vi "IDE_msg_Example_new.vi"() -> ()   [LabVIEW 2020]
uses:
  LabVIEWCode/Subs/ColorText/Code.xctl
  LabVIEWCode/Subs/Console XCtrl/Console_Xctrl.xctl
  LabVIEWCode/Subs/Server XCtrl/Server.xctl
panel:
  in  "Clean":bool
  in  "PC Save":bool
  in  "PC path":path=path "/Users/milandahal/Documents/GitHub/Summer2020/MilanTest/request.py"
  in  "Files":bool
  in  "Server":bool
  in  "Help":bool
  in  "Server":path(xcontrol)=path "/Users/milandahal/Documents/GitHub/Summer2020/LabVIEWCode/Servers/Jens.vi"
  out "REPL":string(xcontrol)="\nTraceback (most recent call last):\n  File \"<stdin>\", line 1\nSyntaxError: invalid syntax\n>>> import hub,utime, ujson\n>>> class request:\n...     def __init__(self):\n...         self.ser = hub.USB_VCP()\n...         self.mbegin=b'msg_start\\n'\n...         self.mend=b'\\nmsg_end\\n'\n...         self.rbegin = b'reply_start '\n...         self.rend = b' reply_end'\n...     def comm(self,payload):\n...         s =  b' '\n...         self.ser.write(self.mbegin + payload + self.mend)\n...         utime.sleep(0.01)\n...         while not(rend in s):\n...             try:\n...                 s = s + self.ser.readline()\n...             except:\n...                 utime.sleep(0.1)\n...         start = len(self.rbegin)+s.find(self.rbegin)\n...         end = s.find(self.rend)\n...         reply = s[start:end]\n...         return reply.decode()\n...     def put(self, headers, url, data):\n...         request= {\"method\": \"put\",\"headers\": ujson.dumps(headers) ,\"url\": url,\"data\": ujson.dumps(data) }\n...         reply=comm(ujson.dumps(request))\n...         utime.sleep(01)\n...         return(reply)        \n...     def post(self, headers, url, data):\n...         request= {\"method\": \"post\",\"headers\": ujson.dumps(headers) ,\"url\": url,\"data\": ujson.dumps(data) }\n...         reply=comm(ujson.dumps(request))\n...         utime.sleep(01)\n...         return(reply)  \n...     def get(self, headers , url):\n...         request= {\"method\": \"get\",\"headers\": ujson.dumps(headers) ,\"url\": url}\n...         reply=comm(ujson.dumps(request))\n...         utime.sleep(01)\n...         return(reply)\n... \n>>> test=request()\n>>> SL_Appkey= \"bvd8X9LweQY9o2eP1NYL-p8mLL9wMAk6YYOnYSiIo0\" \n>>> Headers={\"Accept\":\"application/json\",\"x-ni-api-key\": SL_Appkey }\n>>> Url=\"https://api.systemlinkcloud.com/nitag/v2/tags/test1/values/current\"\n>>> Data={\"value\":{\"type\":\"STRING\",\"value\":\"lol\"}}\n>>> print(reply1)\n{\"timestamp\":\"2020-06-05T14:56:55.375191Z\",\"value\":{\"type\":\"STRING\",\"value\":\"lol\"}}\n>>> key = \"b6fb6cd636d2c3f44a1f7949ff4febf7\"\n>>> city_id = \"7872695\" \n>>> baseurl = \"https://api.openweathermap.org/\"\n>>> url = baseurl + \"data/2.5/weather?id=\" + city_id + \"&appid=\" + key\n>>> reply3= test.get(headers={}, url=url)\nmsg_start\n{\"url\": \"https://api.openweathermap.org/data/2.5/weather?id=7872695&appid=b6fb6cd636d2c3f44a1f7949ff4febf7\", \"headers\": \"{}\", \"method\": \"get\"}\nmsg_end\nb' \\n'\nb' \\nreply_start {\"coord\":{\"lon\":16.21,\"lat\":47.19},\"weather\":[{\"id\":804,\"main\":\"Clouds\",\"description\":\"overcast clouds\",\"icon\":\"04d\"}],\"base\":\"stations\",\"main\":{\"temp\":289.53,\"feels_like\":290.97,\"temp_min\":289.26,\"temp_max\":289.82,\"pressure\":1001,\"humidity\":94},\"wind\":{\"speed\":0.46,\"deg\":71},\"clouds\":{\"all\":100},\"dt\":1591370040,\"sys\":{\"type\":3,\"id\":2007196,\"country\":\"AT\",\"sunrise\":1591326068,\"sunset\":1591382795},\"timezone\":7200,\"id\":7872695,\"name\":\"Olbendorf\",\"cod\":200} reply_end'\n>>> reply_start {\"coord\":{\"lon\":16.21,\"lat\":47.19},\"weather\":[{\"id\":804,\"main\":\"Clouds\",\"description\":\"overcast clouds\",\"icon\":\"04d\"}],\"base\":\"stations\",\"main\":{\"temp\":289.53,\"feels_like\":290.97,\"temp_min\":289.26,\"temp_max\":289.82,\"pressure\":1001,\"humidity\":94},\"wind\":{\"speed\":0.46,\"deg\":71},\"clouds\":{\"all\":100},\"dt\":1591370040,\"sys\":{\"type\":3,\"id\":2007196,\"country\":\"AT\",\"sunrise\":1591326068,\"sunset\":1591382795},\"timezone\":7200,\"id\":7872695,\"name\":\"Olbendorf\",\"cod\":200} reply_end\nTraceback (most recent call last):\n  File \"<stdin>\", line 1\nSyntaxError: invalid syntax\n>>> \n>>> print(reply3)\n{\"coord\":{\"lon\":16.21,\"lat\":47.19},\"weather\":[{\"id\":804,\"main\":\"Clouds\",\"description\":\"overcast clouds\",\"icon\":\"04d\"}],\"base\":\"stations\",\"main\":{\"temp\":289.53,\"feels_like\":290.97,\"temp_min\":289.26,\"temp_max\":289.82,\"pressure\":1001,\"humidity\":94},\"wind\":{\"speed\":0.46,\"deg\":71},\"clouds\":{\"all\":100},\"dt\":1591370040,\"sys\":{\"type\":3,\"id\":2007196,\"country\":\"AT\",\"sunrise\":1591326068,\"sunset\":1591382795},\"timezone\":7200,\"id\":7872695,\"name\":\"Olbendorf\",\"cod\":200}\n>>> import hub,utime, ujson\n>>> class request:\n...     def __init__(self):\n...         self.ser = hub.USB_VCP()\n...         self.mbegin=b'msg_start\\n'\n...         self.mend=b'\\nmsg_end\\n'\n...         self.rbegin = b'reply_start '\n...         self.rend = b' reply_end'\n...     def comm(self,payload):\n...         s =  b' '\n...         self.ser.write(self.mbegin + payload + self.mend)\n...         utime.sleep(0.01)\n...         while not(rend in s):\n...             try:\n...                 s = s + self.ser.readline()\n...             except:\n...                 utime.sleep(0.1)\n...         start = len(self.rbegin)+s.find(self.rbegin)\n...         end = s.find(self.rend)\n...         reply = s[start:end]\n...         return reply.decode()\n...     def put(self, headers, url, data):\n...         request= {\"method\": \"put\",\"headers\": ujson.dumps(headers) ,\"url\": url,\"data\": ujson.dumps(data) }\n...         reply=comm(ujson.dumps(request))\n...         utime.sleep(01)\n...         return(reply)        \n...     def post(self, headers, url, data):\n...         request= {\"method\": \"post\",\"headers\": ujson.dumps(headers) ,\"url\": url,\"data\": ujson.dumps(data) }\n...         reply=comm(ujson.dumps(request))\n...         utime.sleep(01)\n...         return(reply)  \n...     def get(self, headers , url):\n...         request= {\"method\": \"get\",\"headers\": ujson.dumps(headers) ,\"url\": url}\n...         reply=comm(ujson.dumps(request))\n...         utime.sleep(01)\n...         return(reply)\n... \n>>> test=request()\n>>> SL_Appkey= \"bvd8X9LweQY9o2eP1NYL-p8mLL9wMAk6YYOnYSiIo0\" \n>>> Headers={\"Accept\":\"application/json\",\"x-ni-api-key\": SL_Appkey }\n>>> Url=\"https://api.systemlinkcloud.com/nitag/v2/tags/test1/values/current\"\n>>> Data={\"value\":{\"type\":\"STRING\",\"value\":\"lol\"}}\n>>> print(reply1)\n{\"timestamp\":\"2020-06-05T14:56:55.375191Z\",\"value\":{\"type\":\"STRING\",\"value\":\"lol\"}}\n>>> key = \"b6fb6cd636d2c3f44a1f7949ff4febf7\"\n>>> city_id = \"7872695\" \n>>> baseurl = \"https://api.openweathermap.org/\"\n>>> url = baseurl + \"data/2.5/weather?id=\" + city_id + \"&appid=\" + key\n>>> reply3= test.get(headers={}, url=url)\nmsg_start\n{\"url\": \"https://api.openweathermap.org/data/2.5/weather?id=7872695&appid=b6fb6cd636d2c3f44a1f7949ff4febf7\", \"headers\": \"{}\", \"method\": \"get\"}\nmsg_end\nb' \\n'\nb' \\nreply_start {\"coord\":{\"lon\":16.21,\"lat\":47.19},\"weather\":[{\"id\":804,\"main\":\"Clouds\",\"description\":\"overcast clouds\",\"icon\":\"04d\"}],\"base\":\"stations\",\"main\":{\"temp\":289.53,\"feels_like\":290.97,\"temp_min\":289.26,\"temp_max\":289.82,\"pressure\":1001,\"humidity\":94},\"wind\":{\"speed\":0.46,\"deg\":71},\"clouds\":{\"all\":100},\"dt\":1591370040,\"sys\":{\"type\":3,\"id\":2007196,\"country\":\"AT\",\"sunrise\":1591326068,\"sunset\":1591382795},\"timezone\":7200,\"id\":7872695,\"name\":\"Olbendorf\",\"cod\":200} reply_end'\n>>> reply_start {\"coord\":{\"lon\":16.21,\"lat\":47.19},\"weather\":[{\"id\":804,\"main\":\"Clouds\",\"description\":\"overcast clouds\",\"icon\":\"04d\"}],\"base\":\"stations\",\"main\":{\"temp\":289.53,\"feels_like\":290.97,\"temp_min\":289.26,\"temp_max\":289.82,\"pressure\":1001,\"humidity\":94},\"wind\":{\"speed\":0.46,\"deg\":71},\"clouds\":{\"all\":100},\"dt\":1591370040,\"sys\":{\"type\":3,\"id\":2007196,\"country\":\"AT\",\"sunrise\":1591326068,\"sunset\":1591382795},\"timezone\":7200,\"id\":7872695,\"name\":\"Olbendorf\",\"cod\":200} reply_end\nTraceback (most recent call last):\n  File \"<stdin>\", line 1\nSyntaxError: invalid syntax\n>>> print(reply3)\n{\"coord\":{\"lon\":16.21,\"lat\":47.19},\"weather\":[{\"id\":804,\"main\":\"Clouds\",\"description\":\"overcast clouds\",\"icon\":\"04d\"}],\"base\":\"stations\",\"main\":{\"temp\":289.53,\"feels_like\":290.97,\"temp_min\":289.26,\"temp_max\":289.82,\"pressure\":1001,\"humidity\":94},\"wind\":{\"speed\":0.46,\"deg\":71},\"clouds\":{\"all\":100},\"dt\":1591370040,\"sys\":{\"type\":3,\"id\":2007196,\"country\":\"AT\",\"sunrise\":1591326068,\"sunset\":1591382795},\"timezone\":7200,\"id\":7872695,\"name\":\"Olbendorf\",\"cod\":200}\n>>> print(\"something\") \nsomething\n>>> "
  in  "Clear":bool
  in  "Save":bool
  in  "Stop":bool
  in  "Run":bool
  in  "Name":string="code.py"
  in  "Code":string(xcontrol)="import hub,utime, ujson\n\n\n\nclass request:\n    def __init__(self):\n        self.ser = hub.USB_VCP()\n        self.mbegin=b'msg_start\\n'\n        self.mend=b'\\nmsg_end\\n'\n        self.rbegin = b'reply_start '\n        self.rend = b' reply_end'\n    \n    def comm(self,payload):\n        s =  b' '\n        self.ser.write(self.mbegin + payload + self.mend)\n        utime.sleep(0.01)\n        while not(rend in s):\n            try:\n                s = s + self.ser.readline()\n                # print(s)   \n            except:\n                utime.sleep(0.1)\n        start = len(self.rbegin)+s.find(self.rbegin)\n        end = s.find(self.rend)\n        reply = s[start:end]\n        \n        return reply.decode()\n    def put(self, headers, url, data):\n        request= {\"method\": \"put\",\"headers\": ujson.dumps(headers) ,\"url\": url,\"data\": ujson.dumps(data) }\n        reply=comm(ujson.dumps(request))\n        utime.sleep(01)\n        return(reply)        \n    def post(self, headers, url, data):\n        request= {\"method\": \"post\",\"headers\": ujson.dumps(headers) ,\"url\": url,\"data\": ujson.dumps(data) }\n        reply=comm(ujson.dumps(request))\n        utime.sleep(01)\n        return(reply)  \n        \n    def get(self, headers , url):\n        request= {\"method\": \"get\",\"headers\": ujson.dumps(headers) ,\"url\": url}\n        reply=comm(ujson.dumps(request))\n        utime.sleep(01)\n        return(reply)\n        \n\ntest=request()\nSL_Appkey= \"bvd8X9LweQY9o2eP1NYL-p8mLL9wMAk6YYOnYSiIo0\" \nHeaders={\"Accept\":\"application/json\",\"x-ni-api-key\": SL_Appkey }\nUrl=\"https://api.systemlinkcloud.com/nitag/v2/tags/test1/values/current\"\n    \nData={\"value\":{\"type\":\"STRING\",\"value\":\"lol\"}}\n# reply= test.put(headers= Headers , url = Url, data= Data )\n\n\n#reply1=test.get(headers=Headers, url=Url) \n    \n    \nprint(reply1)\n\n\n\n\nkey = \"b6fb6cd636d2c3f44a1f7949ff4febf7\"\n\n# Replace the city id with your city's id\n#Find the entire list of id here http://bulk.openweathermap.org/sample/\n\ncity_id = \"7872695\" # Olbendorf \n\n# base url of the API\nbaseurl = \"https://api.openweathermap.org/\"\n\n# format the baseurl, city and API key into a url\nurl = baseurl + \"data/2.5/weather?id=\" + city_id + \"&appid=\" + key\n\nreply3= test.get(headers={}, url=url)\n\n\n\nprint(reply3)\n\n\nprint(\"something\") \n\n\n\n\n\n\n"
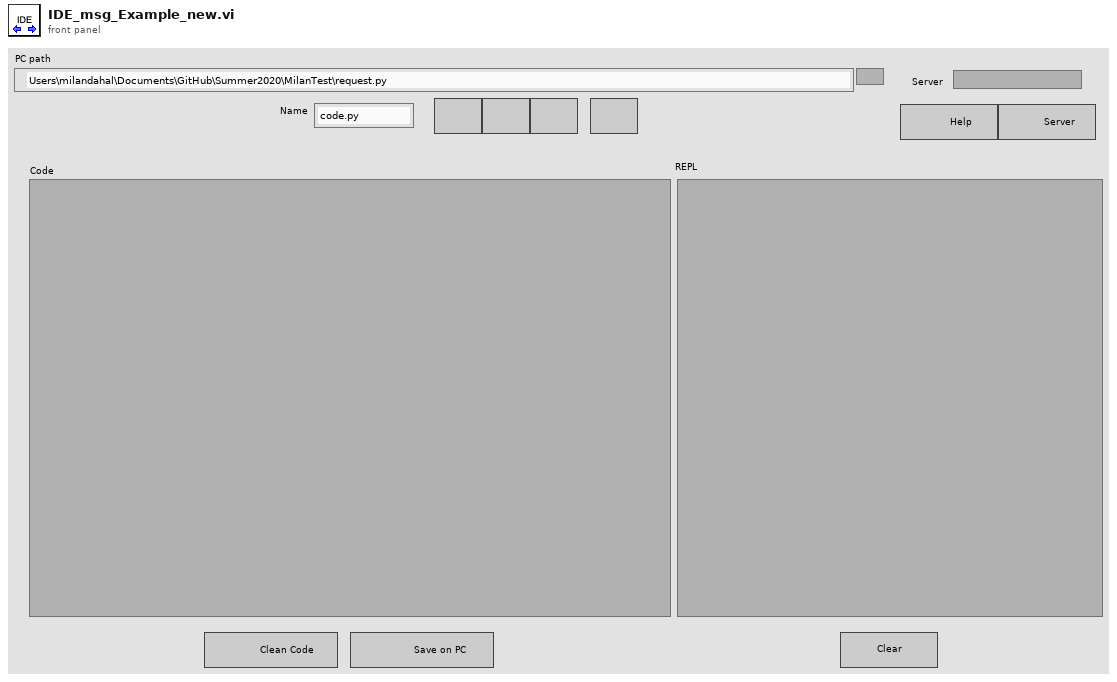
[diagram p1: front panel]
types:
  T1 = cluster{"Quote":u32, "Comment":u32, "Python":u32, "Text":u32, "Triple Quote":u32, "function":u32, "Line numbers":u32, "REPL Err":u32, "REPL Text":u32, "Text Bkgd":u32, "REPL Bkgd":u32}
  T2 = enum8{"Enabled", "Disabled", "Disabled and Grayed Out"}
  T3 = typedef "eventvkey.ctl" = enum16{"ASCII", "Enter", "Return", "Shift", "Ctrl", "Alt", "Cmd", "Opt", "Caps", "NumLock", "Clear", "Break", "Up", "Down", "Left", "Right", "Insert", "Delete", "Home", "End", "PageUp", "PageDown", "Escape", "Help", "Pause", "ScrollLock", "F1", "F2", "F3", "F4", "F5", "F6", "F7", "F8", "F9", "F10", "F11", "F12", "F13", "F14", "F15", "F16", "F17", "F18", "F19", "F20", "F21", "F22", "F23", "F24", "Play", "VolumeUp", "VolumeDown", "Mute", "Two Byte Char"}
  T4 = cluster{"Shift":bool, "Ctrl":bool, "Alt":bool, "Cmd":bool, "Opt":bool}
  T5 = cluster{"Char":i16, "VKey":T3, "PlatMods":cluster{"Shift":bool, "Ctrl":bool, "Alt":bool, "Cmd":bool, "Opt":bool}}
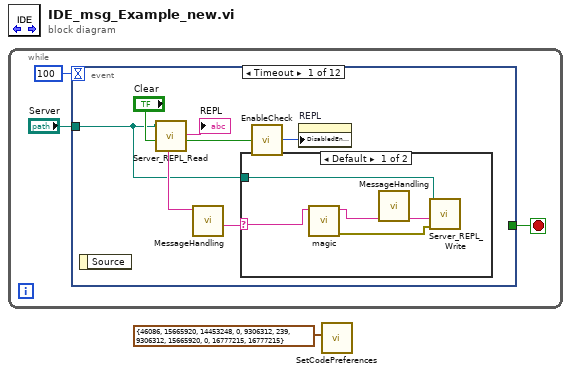
[diagram p0: block diagram]
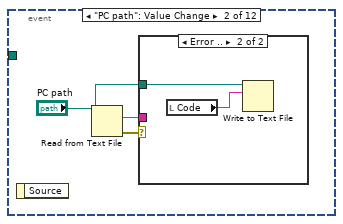
[diagram p3: hidden frame]
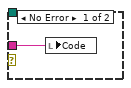
[diagram p4: hidden frame]
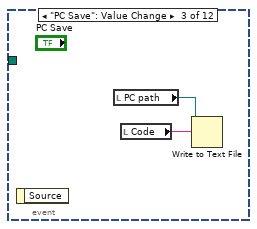
[diagram p5: hidden frame]
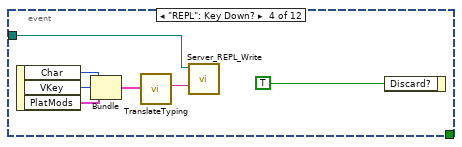
[diagram p6: hidden frame]
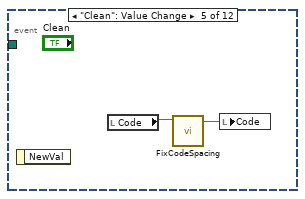
[diagram p7: hidden frame]
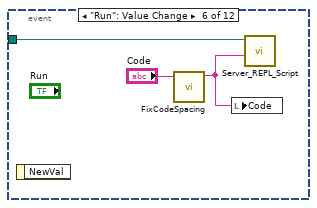
[diagram p8: hidden frame]
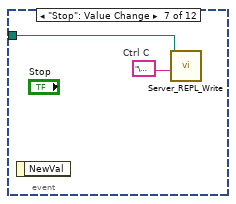
[diagram p9: hidden frame]
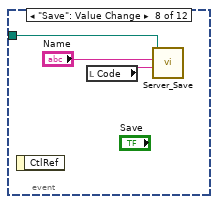
[diagram p10: hidden frame]
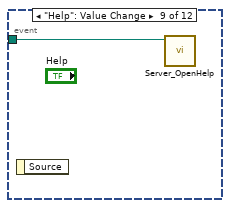
[diagram p11: hidden frame]
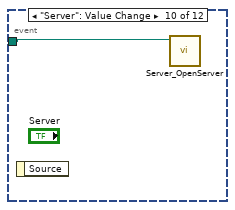
[diagram p12: hidden frame]
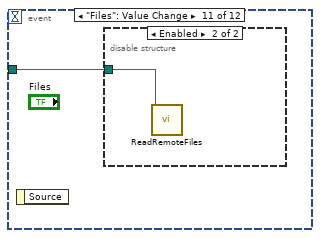
[diagram p13: hidden frame]
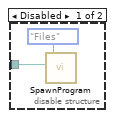
[diagram p14: hidden frame]
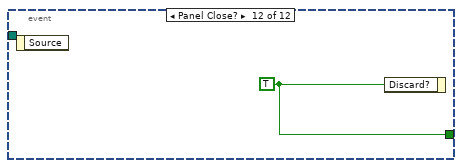
[diagram p15: hidden frame]
diagram:
  n1 = while {
    stop <- w3 stop-if-true
    n2 = event shown="[0] Timeout" {
      selector: _ -> [_ _ _ _ _ _ _ _ _ _ _ _]
      dyn-events: _ -> [_ _ _ _ _ _ _ _ _ _ _ _]
      timeout: 100 -> [_ _ _ _ _ _ _ _ _ _ _ _]
      tunnel: [_ _ _ _ _ _ _ _ _ _ _ w47] -> w3
      tunnel: "Server" -> [w5 _ _ w24 _ w34 w36 w38 w41 w42 w43 _]
      event Timeout {
        n3 = event-data() -> ()  [unwired: 1 in, 1 out]
        n4 = call "Server_REPL_Read.vi"("Clear"="Clear", "Server"=w5) -> ("Running?"=w9:bool, "REPL"=w7:string)  [unwired: 7 in, 1 out]
        "REPL" <- w7
        n5 = call "MessageHandling.vi"("REPL"=w7) -> ("New Message"=w6:string)  [unwired: 7 in, 3 out]
        n6 = case shown="Default" w6 {
          selector: w6 -> [w13 _]
          tunnel: w5 -> [w15 _]
          frame Default {
            n7 = call "magic.vi"("payload"=w13) -> ("error out"=w11:errorcluster, "body"=w12:string)  [unwired: 9 in]
            n8 = call "MessageHandling.vi"("Reply"=w12) -> ("New Reply"=w14:string)  [unwired: 7 in, 3 out]
            n9 = call "Server_REPL_Write.vi"("error in (no error)"=w11, "Code"=w14, "Server"=w15) -> ()  [unwired: 8 in, 1 out]
          }
          frame "" {
          }
        }
        n10 = call "EnableCheck.vi"("Enable?"=w9) -> ("Enum"=w10:T2)
        n11 = property on="REPL" class="Console_Xctrl (strict)"("DisabledEnum"=w10) -> ()  [unwired: 2 in, 2 out]
      }
      event "PC path": Value Change {
        n12 = event-data() -> ()  [unwired: 1 in, 1 out]
        n13 = Read from Text File(file (use dialog)="PC path") -> (text=w17:string, error out=w18:errorcluster)  [unwired: 3 in, 2 out]
        n14 = case shown="Error .." w18 {
          tunnel: w17 -> [w19 _]
          tunnel: "PC path" -> [_ w21]
          frame No Error {
            n15 = local write "Code"(w19) -> ()
          }
          frame Error {
            n16 = local read "Code"() -> (w20:string)
            n17 = Write to Text File(file (use dialog)=w21, text=w20) -> ()  [unwired: 2 in, 3 out]
          }
        }
      }
      event "PC Save": Value Change {
        n18 = event-data() -> ()  [unwired: 1 in, 1 out]
        n19 = local read "PC path"() -> (w23:path)
        n20 = local read "Code"() -> (w22:string)
        n21 = Write to Text File(file (use dialog)=w23, text=w22) -> ()  [unwired: 2 in, 3 out]
      }
      event "REPL": Key Down? {
        n22 = event-data() -> ("Char"=w29:i16, "VKey"=w28:T3, "PlatMods"=w26:T4)  [unwired: 1 in]
        n23 = Bundle("Char"=w29, "VKey"=w28, "PlatMods"=w26) -> (w30:T5)  [unwired: 1 in]
        n24 = call "TranslateTyping.vi"("Cluster"=w30) -> ("key"=w25:string)  [unwired: 10 in]
        n25 = call "Server_REPL_Write.vi"("Code"=w25, "Server"=w24) -> ()  [unwired: 9 in, 1 out]
        n26 = event-data("Discard?"=TRUE) -> ()  [unwired: 1 in, 1 out]
      }
      event "Clean": Value Change {
        n27 = event-data() -> ()  [unwired: 1 in, 1 out]
        n28 = local read "Code"() -> (w31:string)
        n29 = call "FixCodeSpacing.vi"("Code"=w31) -> ("Cleaned"=w32:string)  [unwired: 10 in]
        n30 = local write "Code"(w32) -> ()
      }
      event "Run": Value Change {
        n31 = event-data() -> ()  [unwired: 1 in, 1 out]
        n32 = call "FixCodeSpacing.vi"("Code"="Code") -> ("Cleaned"=w33:string)  [unwired: 10 in]
        n33 = local write "Code"(w33) -> ()
        n34 = call "Server_REPL_Script.vi"("Code"=w33, "Server"=w34) -> ()  [unwired: 9 in, 1 out]
      }
      event "Stop": Value Change {
        w37 = "\u0003"  # Ctrl C
        n35 = event-data() -> ()  [unwired: 1 in, 1 out]
        n36 = call "Server_REPL_Write.vi"("Code"=w37, "Server"=w36) -> ()  [unwired: 9 in, 1 out]
      }
      event "Save": Value Change {
        n37 = event-data() -> ()  [unwired: 1 in, 1 out]
        n38 = local read "Code"() -> (w40:string)
        n39 = call "Server_Save.vi"("Code"=w40, "Name"="Name", "Server"=w38) -> ()  [unwired: 8 in, 1 out]
      }
      event "Help": Value Change {
        n40 = event-data() -> ()  [unwired: 1 in, 1 out]
        n41 = call "Server_OpenHelp.vi"("Server"=w41) -> ()  [unwired: 10 in, 1 out]
      }
      event "Server": Value Change {
        n42 = event-data() -> ()  [unwired: 1 in, 1 out]
        n43 = call "Server_OpenServer.vi"("Server"=w42) -> ()  [unwired: 10 in, 1 out]
      }
      event "Files": Value Change {
        n44 = event-data() -> ()  [unwired: 1 in, 1 out]
        n45 = disable-structure shown="Enabled" {
          disable-tunnel: w43 -> [w44 w46]
          frame Disabled {
            n46 = call "SpawnProgram.vi"("Server"=w44, "Dialog"=enum16{"Help", "Files"}."Files") -> ()  [unwired: 10 in]
          }
          frame Enabled {
            n47 = call "ReadRemoteFiles.vi"("Server"=w46) -> ()  [unwired: 11 in]
          }
        }
      }
      event Panel Close? {
        w47 = TRUE ("Discard?")
        n48 = event-data() -> ()  [unwired: 1 in, 1 out]
        n49 = event-data("Discard?"=w47) -> ()  [unwired: 1 in, 1 out]
      }
    }
  }
  n50 = call "SetCodePreferences.vi"("Color choices"=T1 {"Quote"=46086, "Comment"=15665920, "Python"=14453248, "Text"=0, "Triple Quote"=9306312, "function"=239, "Line numbers"=9306312, "REPL Err"=15665920, "REPL Text"=0, "Text Bkgd"=16777215, "REPL Bkgd"=16777215}) -> ()  [unwired: 11 in]
